vi "Init.vi"(8 "error in":errorcluster, 11 "Cell View in":refnum<class "Cell View.lvclass">) -> (0 "error out":errorcluster, 3 "Cell View out":refnum<class "Cell View.lvclass">)   [LabVIEW 2024, in "Cell View.lvclass"]
uses:
  Cell View.lvclass
  Cell View.lvclass/Cell View.ctl
  D:/git/Sourcegrid-LabVIEW/dll/SourceGrid.dll
  dll/SourceGrid.dll
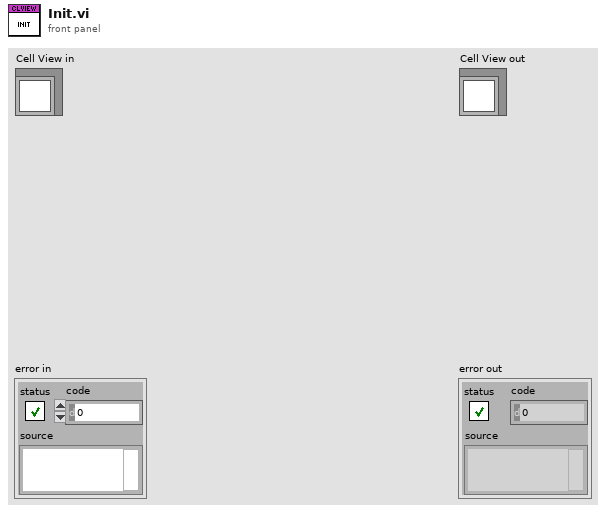
[diagram p1: front panel]
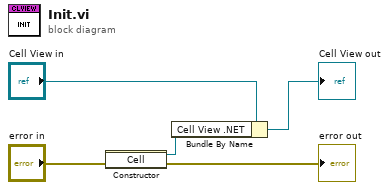
[diagram p0: block diagram]
diagram:
  n1 = constructor class="Cell"(error in="error in") -> (reference out=w1:refnum<k24>, error out=→"error out":errorcluster)  [unwired: 2 in, 1 out]
  n2 = Bundle By Name(cluster="Cell View in", "Cell View .NET"=w1) -> (→"Cell View out":refnum<class "Cell View.lvclass">)
